vi "Editor.vi"(9 "Editor Events":T1, 11 "Parser Settings In":refnum<class "Parser Settings.lvclass">) -> (3 "Parser Settings Out":refnum<class "Parser Settings.lvclass">)   [LabVIEW 2023, in "VIDoc Parsing.lvlib" / "Parser Settings.lvclass"]
uses:
  Parser Settings.lvclass
  Draw Controls Cluster.ctl
  Draw Option Enum.ctl
  Editors/VIDoc Editor/Editor Events Cluster.ctl
  Parser Settings.lvclass/Parser Settings.ctl
  Editors/VIDoc Editor/VIDocEditor.lvclass
panel:
  in  "Bookmarks":cluster{"Term":string, "Bookmarks":string[]}[](array[cluster])
  in  "Max Control Recursion Depth":i32
  in  "Draw Controls":T2
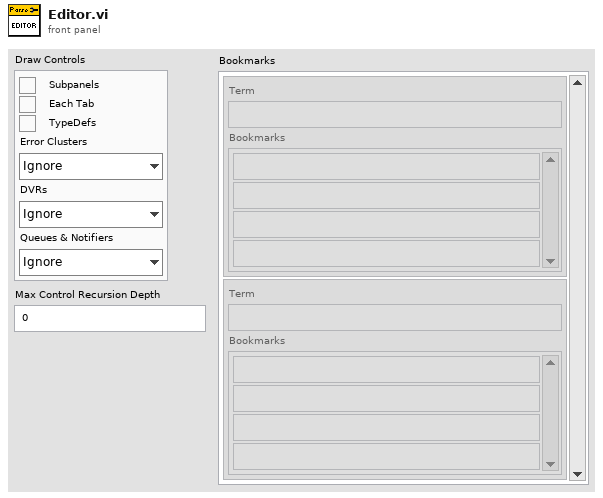
[diagram p1: front panel]
types:
  T1 = typedef "VIDocEditor.lvclass/Editor Events Cluster.ctl" = cluster{"Close":refnum<user-event>, "Revert":refnum<user-event>, "Save":refnum<user-event>, "Changes?":refnum<user-event>}
  T2 = typedef "VIDoc Parsing.lvlib/Parser Settings.lvclass/Draw Controls Cluster.ctl" = cluster{"Subpanels":bool, "Tabs":bool, "TypeDefs":bool, "Error Clusters":T3, "DVRs":T3, "Queues & Notifiers":T3}
  T3 = typedef "VIDoc Parsing.lvlib/Parser Settings.lvclass/Draw Option Enum.ctl" = enum16{"Ignore", "Draw", "Draw + Contents"}
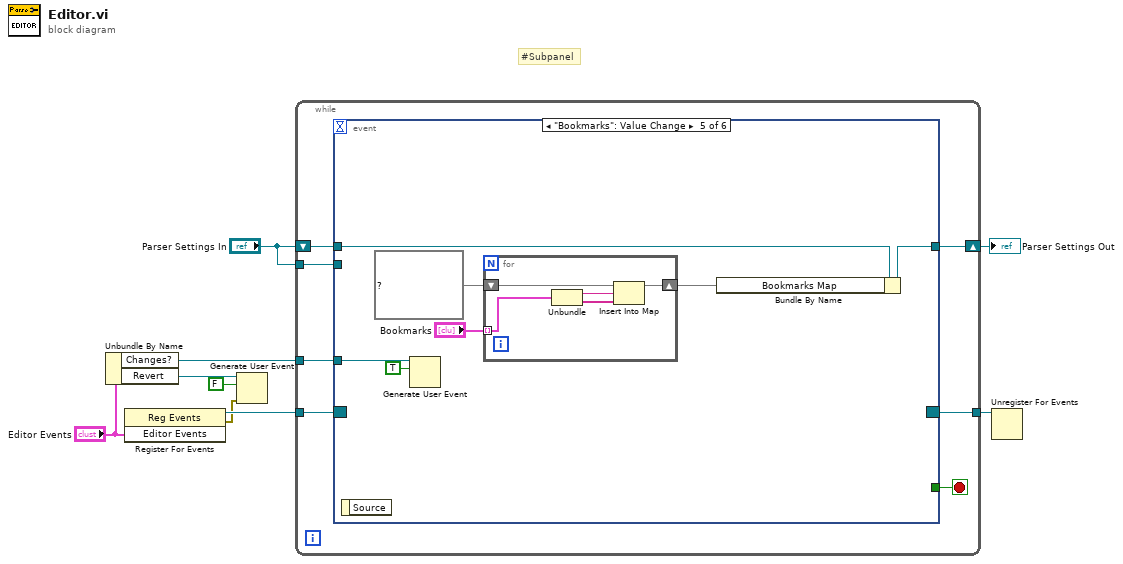
[diagram p0: block diagram]
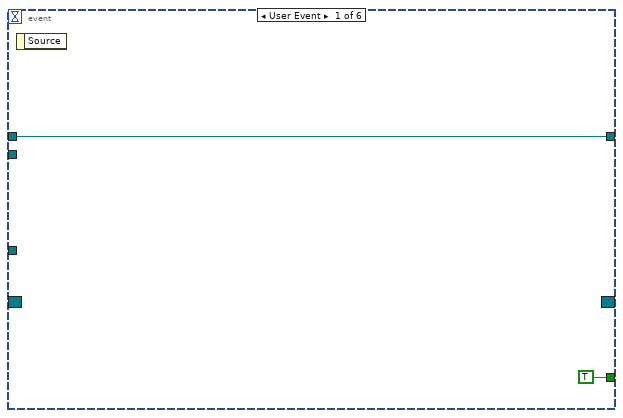
[diagram p2: hidden frame]
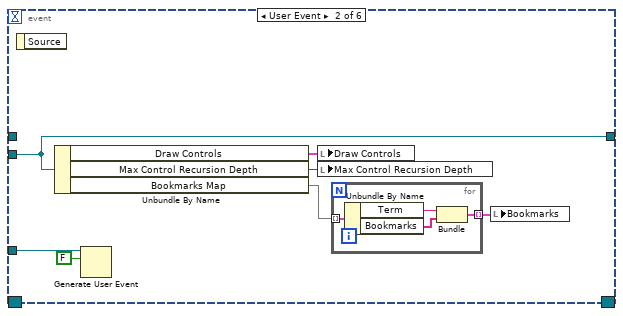
[diagram p3: hidden frame]
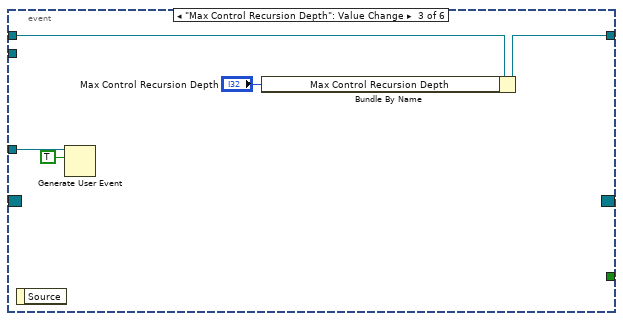
[diagram p4: hidden frame]
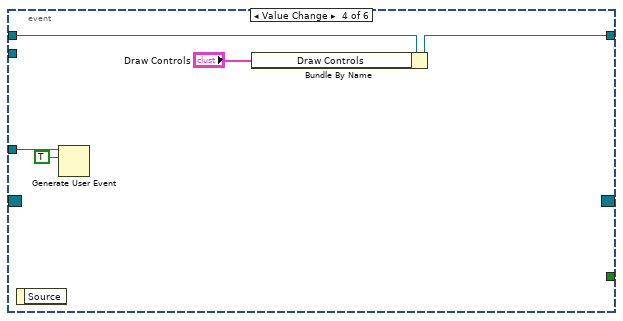
[diagram p5: hidden frame]
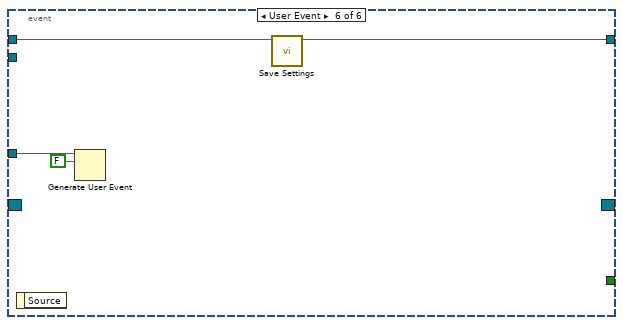
[diagram p6: hidden frame]
diagram:
  # "#Subpanel"
  n1 = Unbundle By Name("Editor Events") -> ("Changes?"=w1:refnum<user-event>, "Revert"=w4:refnum<user-event>)
  n2 = register-events("Editor Events") -> (reference out=w9:refnum<event-registration>, error out=w2:errorcluster)  [unwired: 2 in]
  n3 = Generate User Event(user event=w4, event data cluster=FALSE ("event data"), error in=w2) -> ()  [unwired: 1 in, 2 out]
  n4 = while {
    shift-right: [w14] -> w7
    shift-left: "Parser Settings In" -> [w16]
    tunnel: w9 -> [w15]
    tunnel: [w12] -> w8
    tunnel: "Parser Settings In" -> [w11]
    tunnel: w1 -> [w10]
    stop <- w13 stop-if-true
    n5 = event shown="[4] \"Bookmarks\": Value Change" {
      selector: w15 -> [_ _ _ _ _ _]
      dyn-events: [_ _ _ _ _ _] -> w12
      timeout: _ -> [_ _ _ _ _ _]
      tunnel: w16 -> [w18 _ w34 w39 w46 w54]
      tunnel: [w18 w25 w33 w38 w45 w55] -> w14
      tunnel: [TRUE _ _ _ _ _] -> w13
      tunnel: w11 -> [_ w25 _ _ _ _]
      tunnel: w10 -> [_ w21 w30 w35 w44 w52]
      event User Event {
        n6 = event-data() -> ()  [unwired: 1 in, 1 out]
      }
      event User Event {
        n7 = event-data() -> ()  [unwired: 1 in, 1 out]
        n8 = Unbundle By Name(w25) -> ("Draw Controls"=w23:T2, "Max Control Recursion Depth"=w24:i32, "Bookmarks Map"=w20:map{string, string[]})
        n9 = Generate User Event(user event=w21, event data cluster=FALSE ("event data")) -> ()  [unwired: 2 in, 2 out]
        n10 = local write "Draw Controls"(w23) -> ()
        n11 = local write "Max Control Recursion Depth"(w24) -> ()
        n12 = for {
          tunnel: w20 -> [w29] mode=indexing
          tunnel: [w26] -> w19 mode=indexing
          n13 = Unbundle By Name(w29) -> ("Term"=w28:string, "Bookmarks"=w27:string[])
          n14 = Bundle("Term"=w28, "Bookmarks"=w27) -> (w26:cluster{"Term":string, "Bookmarks":string[]})  [unwired: 1 in]
        }
        n15 = local write "Bookmarks"(w19) -> ()
      }
      event "Max Control Recursion Depth": Value Change {
        n16 = event-data() -> ()  [unwired: 1 in, 1 out]
        n17 = Generate User Event(user event=w30, event data cluster=TRUE ("event data")) -> ()  [unwired: 2 in, 2 out]
        n18 = Bundle By Name(cluster=w34, "Max Control Recursion Depth"="Max Control Recursion Depth") -> (w33:refnum<class "Parser Settings.lvclass">)
      }
      event Value Change {
        n19 = event-data() -> ()  [unwired: 1 in, 1 out]
        n20 = Generate User Event(user event=w35, event data cluster=TRUE ("event data")) -> ()  [unwired: 2 in, 2 out]
        n21 = Bundle By Name(cluster=w39, "Draw Controls"="Draw Controls") -> (w38:refnum<class "Parser Settings.lvclass">)
      }
      event "Bookmarks": Value Change {
        n22 = event-data() -> ()  [unwired: 1 in, 1 out]
        n23 = Generate User Event(user event=w44, event data cluster=TRUE ("event data")) -> ()  [unwired: 2 in, 2 out]
        n24 = for {
          shift-right: [w50] -> w41
          shift-left: map{string, string[]} {} ("Parser Settings.Bookmarks Map") -> [w51]
          tunnel: "Bookmarks" -> [w49] mode=indexing
          n25 = Unbundle(w49) -> ("Term"=w48:string, "Bookmarks"=w47:string[])
          n26 = Insert Into Map(map in=w51, key=w48, value=w47) -> (map out=w50:map{string, string[]})  [unwired: 2 out]
        }
        n27 = Bundle By Name(cluster=w46, "Bookmarks Map"=w41) -> (w45:refnum<class "Parser Settings.lvclass">)
      }
      event User Event {
        n28 = event-data() -> ()  [unwired: 1 in, 1 out]
        n29 = Generate User Event(user event=w52, event data cluster=FALSE ("event data")) -> ()  [unwired: 2 in, 2 out]
        n30 = call-dynamic "Save Settings.vi"("Parser Settings In"=w54) -> ("Parser Settings Out"=w55:refnum<class "Parser Settings.lvclass">)  [unwired: 9 in, 1 out]
      }
    }
  }
  "Parser Settings Out" <- w7
  n31 = Unregister For Events(event registration refnum=w8) -> ()  [unwired: 1 in, 1 out]
